vi "Q.Build Element.vi"(8 "Data2":variant, 9 "Data1":variant, 10 "Sub":string, 11 "Cmd":string) -> (3 "Q.Element":T1)   [LabVIEW 2024, in "EQMF.lvlib" / "Queue Utils.lvlib"]
uses:
  Queue Utils.lvlib
  Q.Element.ctl
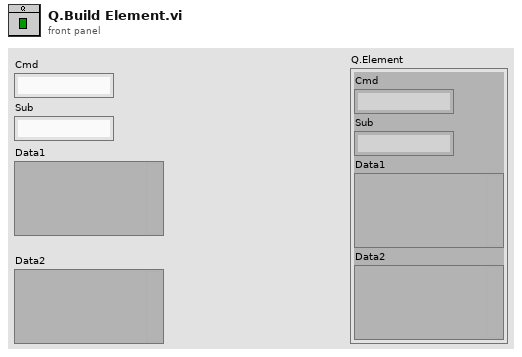
[diagram p1: front panel]
types:
  T1 = typedef "EQMF.lvlib/Queue Utils.lvlib/Q.Element.ctl" = cluster{"Cmd":string, "Sub":string, "Data1":variant, "Data2":variant}
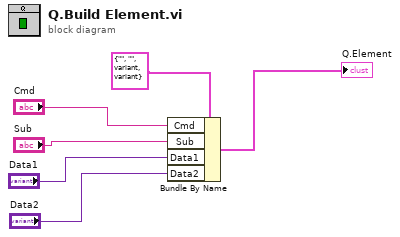
[diagram p0: block diagram]
diagram:
  n1 = Bundle By Name(cluster=T1 {"Cmd"="", "Sub"="", "Data1"=variant, "Data2"=variant} ("Q.Element"), "Cmd"="Cmd", "Sub"="Sub", "Data1"="Data1", "Data2"="Data2") -> (→"Q.Element":T1)
